vi "MiniBot Release.vi"(10 "Limit Switch":bool, 11 "Mini Bot Trigger":bool) -> (3 "Minibot Release Motor Output":dbl)   [LabVIEW 2011]
uses:
  Robot Global Data.vi
panel:
  out "Minibot Release State":dbl
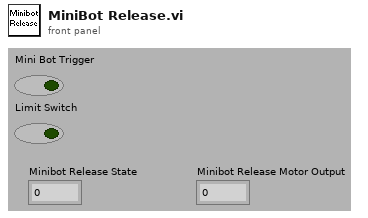
[diagram p1: front panel]
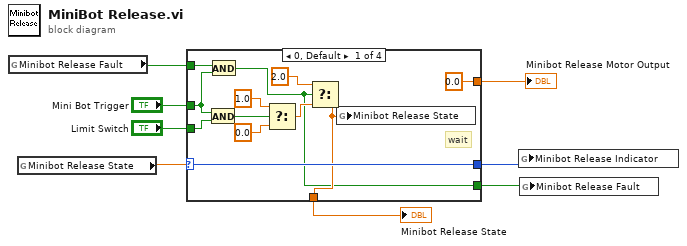
[diagram p0: block diagram]
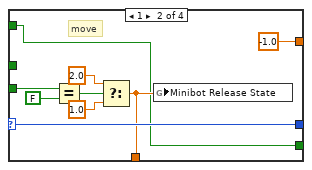
[diagram p2: hidden frame]
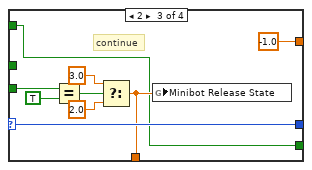
[diagram p3: hidden frame]
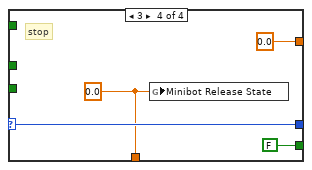
[diagram p4: hidden frame]
diagram:
  n1 = global read "Robot Global Data.vi" "Minibot Release Fault"() -> (w2:bool)
  n2 = global read "Robot Global Data.vi" "Minibot Release State"() -> (w3:dbl)
  n3 = case shown="0, Default" w3 {
    selector: w3 -> [w15 w23 w32 w42]
    tunnel: "Mini Bot Trigger" -> [w12 _ _ _]
    tunnel: "Limit Switch" -> [w20 w25 w34 _]
    tunnel: [0.0 -1.0 -1.0 0.0] -> w6
    tunnel: [w15 w23 w32 w42] -> w5
    tunnel: w2 -> [w13 w21 w30 _]
    tunnel: [w10 w22 w31 w40] -> w4
    tunnel: [w9 w21 w30 FALSE ("Minibot Release Fault")] -> w1
    frame 0, Default {
      # "wait"
      n4 = And(x=w12, y=w20) -> (x .and. y?=w19:bool)
      n5 = And(x=w13, y=w12) -> (x .and. y?=w9:bool)
      n6 = Select(t=1.0, s=w19, f=0.0) -> (s? t:f=w14:dbl)
      n7 = Select(t=2.0, s=w9, f=w14) -> (s? t:f=w10:dbl)
      n8 = global write "Robot Global Data.vi" "Minibot Release State"(w10) -> ()
    }
    frame 1 {
      # "move"
      n9 = Equal?(x=w25, y=FALSE) -> (x = y?=w26:bool)
      n10 = Select(t=2.0, s=w26, f=1.0) -> (s? t:f=w22:dbl)
      n11 = global write "Robot Global Data.vi" "Minibot Release State"(w22) -> ()
    }
    frame 2 {
      # "continue"
      n12 = Equal?(x=w34, y=TRUE) -> (x = y?=w35:bool)
      n13 = Select(t=3.0, s=w35, f=2.0) -> (s? t:f=w31:dbl)
      n14 = global write "Robot Global Data.vi" "Minibot Release State"(w31) -> ()
    }
    frame 3 {
      w40 = 0.0 ("Minibot Release State")
      # "stop"
      n15 = global write "Robot Global Data.vi" "Minibot Release State"(w40) -> ()
    }
  }
  "Minibot Release State" <- w4
  "Minibot Release Motor Output" <- w6
  n16 = global write "Robot Global Data.vi" "Minibot Release Indicator"(w5) -> ()
  n17 = global write "Robot Global Data.vi" "Minibot Release Fault"(w1) -> ()
